vi "take and write data.vi"(9 "y":dbl, 10 "Path":path, 11 "Current position (units)":dbl) -> ()   [LabVIEW 2011]
uses:
  <vilib>/Utility/file.llb/Write To Spreadsheet File (DBL).vi
panel:
  out "array":i32[](array[numeric])
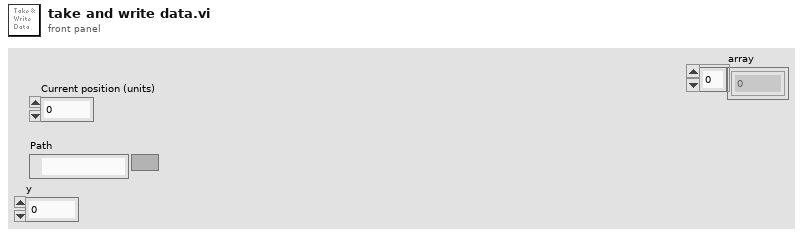
[diagram p1: front panel]
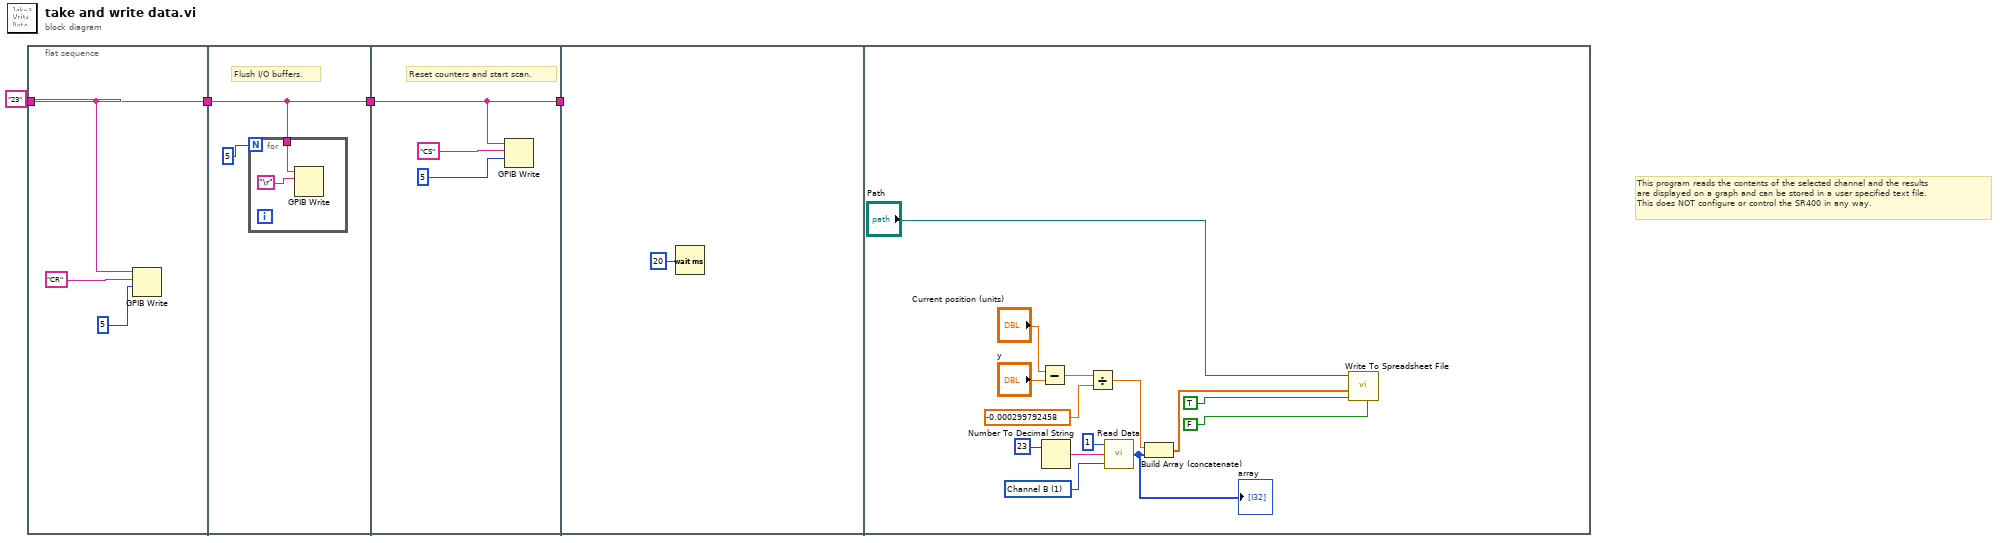
[diagram p0: block diagram]
diagram:
  # "This program reads the contents of the selected channel and the results\nare displayed on a graph and can be stored in a user specified text file.\nThis does NOT configure or control the SR400 in any way."
  n1 = flat-sequence {
    tunnel: "23" ("GPIB Address") -> [w5]
    tunnel: [w5] -> w2
    tunnel: [w9] -> w4
    tunnel: w2 -> [w9]
    tunnel: w4 -> [w12]
    tunnel: [w12] -> w1
    tunnel: w1 -> [_]
    frame #0 {
      n2 = GPIB Write(0:w5, 1:"CR", 2:i16 5 ("mode (0)")) -> ()  [unwired: 2 in, 2 out]
    }
    frame #1 {
      # "Flush I/O buffers."
      n3 = for {
        N: 5 -> [_]
        tunnel: w9 -> [w10]
        n4 = GPIB Write(0:w10, 1:"\r") -> ()  [unwired: 3 in, 2 out]
      }
    }
    frame #2 {
      # "Reset counters and start scan."
      n5 = GPIB Write(0:w12, 1:"CS", 2:i16 5 ("mode (0)")) -> ()  [unwired: 2 in, 2 out]
    }
    frame #3 {
      n6 = Wait (ms)(milliseconds to wait=u32 20) -> ()  [unwired: 1 out]
    }
    frame #4 {
      w22 = u16 1 items=["Channel A", "Channel B"] ("Select Channel")
      n7 = Subtract(x="Current position (units)", y="y") -> (x-y=w18:dbl)
      n8 = Number To Decimal String(number=23 ("GPIB Address")) -> (decimal integer string=w24:string)  [unwired: 1 in]
      n9 = Divide(x=w18, y=-0.000299792458) -> (x/y=w19:dbl)
      n10 = call "Read Data.vi"("Channel Number"=w22, "GPIB Address"=w24, "Number of Datapoints"=1) -> ("Data"=w16:i32[])
      "array" <- w16
      n11 = Build Array (concatenate)(w19, w16) -> (w26:dbl[])
      n12 = call-poly <vilib>:"Write To Spreadsheet File.vi"("transpose? (no:F)"=FALSE, "append to file? (new file:F)"=TRUE, "1D data"=w26, "file path (dialog if empty)"="Path") -> ()  [unwired: 4 in, 1 out]
    }
  }
